vi "chronus_helper.vi"(4 "ms between iterations":i32, 5 "iteration number":i32) -> (0 "time (s)":dbl, 1 "time (ms)":dbl, 2 "write to file":bool)   [LabVIEW 2010]
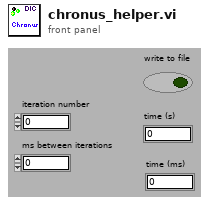
[diagram p1: front panel]
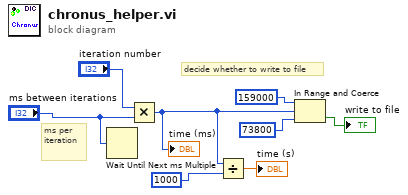
[diagram p0: block diagram]
diagram:
  # "decide whether to write to file"
  # "ms per iteration"
  n1 = Wait Until Next ms Multiple(millisecond multiple="ms between iterations") -> ()  [unwired: 1 out]
  n2 = Multiply(x="iteration number", y="ms between iterations") -> (x*y=w6:i32)
  "time (ms)" <- w6
  n3 = Divide(x=w6, y=1000) -> (x/y=→"time (s)":dbl)
  n4 = In Range and Coerce(upper limit=159000, x=w6, lower limit=73800) -> (In Range?=→"write to file":bool)  [unwired: 1 out]
